vi "R_W_Heater_Setup.vi"(2 "Mode":enum16{"Load from File", "Save to File"}(ring), 3 "Setpoints In":T1[](array[typedef])) -> (1 "Setpoints Out":T1[](array[typedef]))   [LabVIEW 2010]
uses:
  Heater_Setpoint.ctl
  Anemometry/Anemometry Sub Vis/Globals/Constants_global.vi
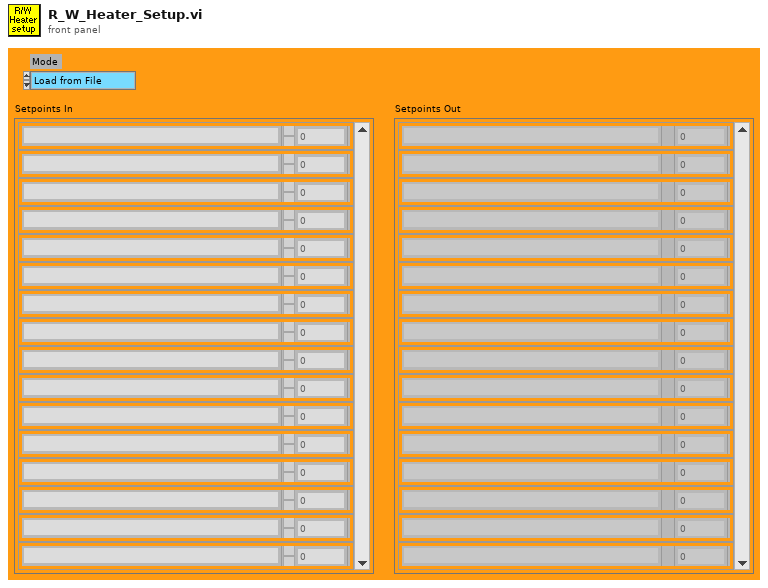
[diagram p1: front panel]
types:
  T1 = typedef "Heater_Setpoint.ctl" = cluster{"Ch Name":string, "Setpoint":dbl}
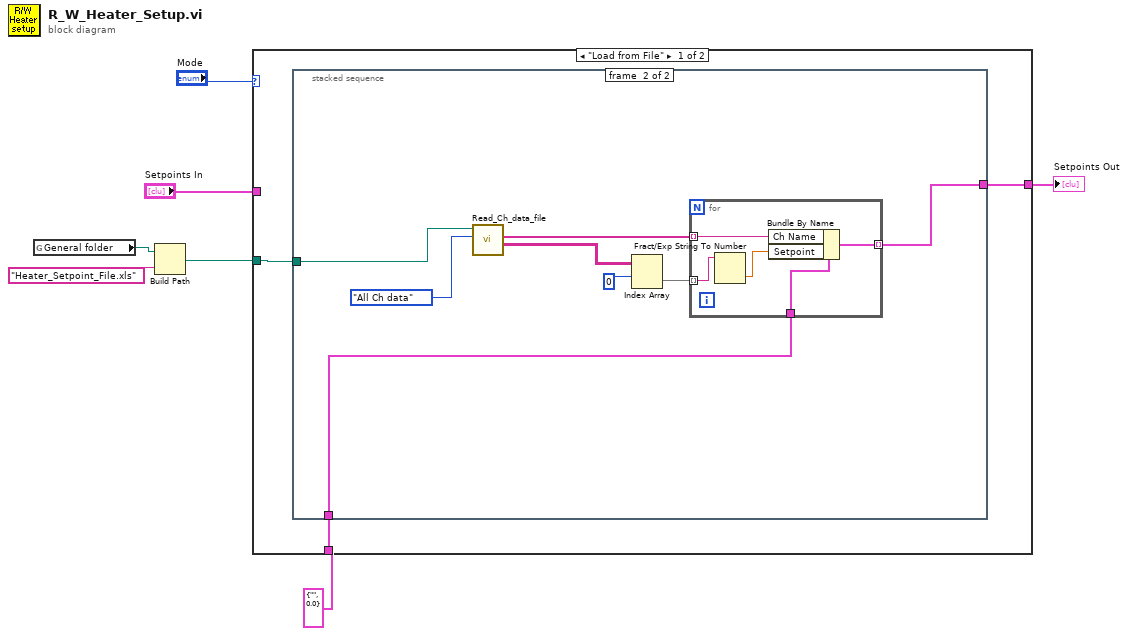
[diagram p0: block diagram]
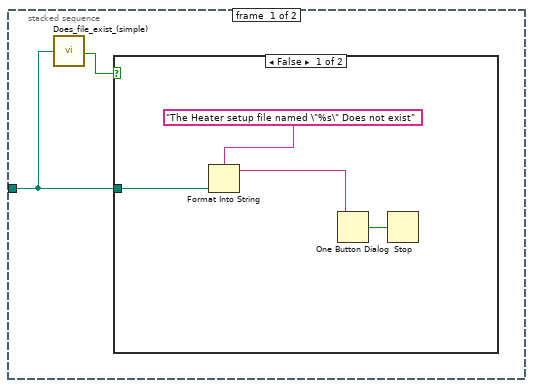
[diagram p2: hidden frame]
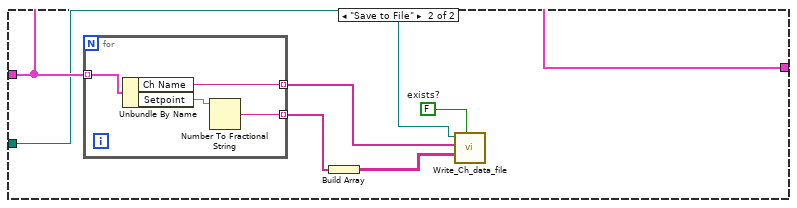
[diagram p4: hidden frame]
diagram:
  n1 = global read "Constants_global.vi" "General folder"() -> (w3:path)
  n2 = Build Path(base path=w3, name or relative path="Heater_Setpoint_File.xls") -> (appended path=w1:path)
  n3 = case shown="\"Load from File\"" "Mode" {
    tunnel: w1 -> [w8 w30]
    tunnel: T1 {"Ch Name"="", "Setpoint"=0.0} ("Cluster") -> [w10 _]
    tunnel: [w9 w31] -> w5
    tunnel: "Setpoints In" -> [_ w31]
    frame "Load from File" {
      n4 = stacked-sequence {
        tunnel: w8 -> [w11 w19]
        tunnel: w10 -> [_ w23]
        tunnel: [_ w21] -> w9
        frame #0 {
          n5 = call "Does_file_exist_(simple).vi"("Pathname"=w11) -> ("exists?"=w12:bool)
          n6 = case shown="False" w12 {
            tunnel: w11 -> [w16 _]
            frame False {
              n7 = Format Into String(format string="The Heater setup file named \"%s\" Does not exist" ("Format String"), w16) -> (resulting string=w15:string)  [unwired: 2 in, 1 out]
              n8 = One Button Dialog(message=w15) -> (true=w13:bool)  [unwired: 1 out]
              n9 = Stop(stop? (T)=w13) -> ()
            }
            frame True {
            }
          }
        }
        frame #1 {
          n10 = call "Read_Ch_data_file.vi"("Output"=enum16{"All Ch data", "The last few rows"}."All Ch data", "Filename"=w19) -> ("Channel Values"=w17:string[][], "Merged Channels"=w18:string[])  [unwired: 3 in, 3 out]
          n11 = Index Array(array=w17, index (row)=0 ("Index")) -> (element=w22:string[])  [unwired: 1 in]
          n12 = for {
            tunnel: w23 -> [w29]
            tunnel: w18 -> [w28] mode=indexing
            tunnel: w22 -> [w27] mode=indexing
            tunnel: [w25] -> w21 mode=indexing
            n13 = Fract/Exp String To Number(string=w27) -> (number=w26:dbl)  [unwired: 4 out]
            n14 = Bundle By Name(cluster=w29, "Ch Name"=w28, "Setpoint"=w26) -> (w25:T1)
          }
        }
      }
    }
    frame "Save to File" {
      w35 = FALSE  # exists?
      n15 = for {
        tunnel: w31 -> [w39] mode=indexing
        tunnel: [w37] -> w33 mode=indexing
        tunnel: [w36] -> w32 mode=indexing
        n16 = Unbundle By Name(w39) -> ("Ch Name"=w36:string, "Setpoint"=w38:dbl)
        n17 = Number To Fractional String(number=w38) -> (F-format string=w37:string)  [unwired: 3 out]
      }
      n18 = Build Array(w33) -> (w34:string[][])
      n19 = call "Write_Ch_data_file.vi"("exists?"=w35, "Channel Values"=w34, "Channel names"=w32, "Filename"=w30) -> ()  [unwired: 4 in, 4 out]
    }
  }
  "Setpoints Out" <- w5
